vi "Cleanup.vi"(8 "error in (no error)":errorcluster, 11 "TCP_Streamer_Subscriber in":refnum<class "TCP_Streamer_Subscriber.lvclass">) -> (0 "error out":errorcluster, 3 "TCP_Streamer_Subscriber out":refnum<class "TCP_Streamer_Subscriber.lvclass">)   [LabVIEW 2021, in "TCP_Streamer_Subscriber.lvclass"]
uses:
  TCP_Streamer_Subscriber.lvclass
  TCP_Streamer_Subscriber.lvclass/TCP_Streamer_Subscriber.ctl
  Typedef/State.ctl
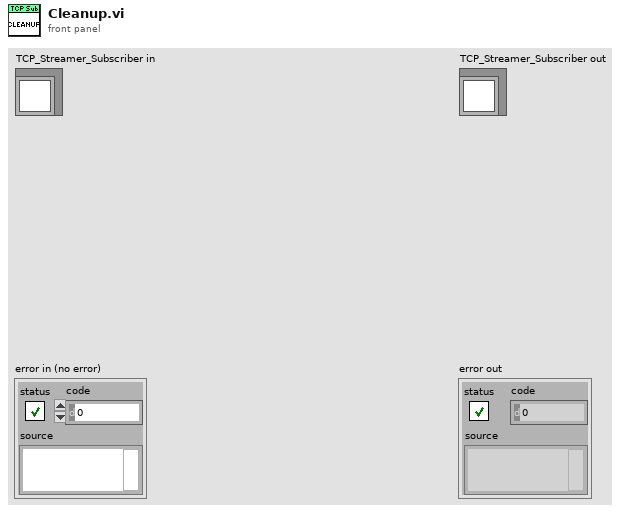
[diagram p1: front panel]
types:
  T1 = typedef "TCP_Streamer_Subscriber.lvclass/State.ctl" = enum16{"Stopped", "Connecting", "Receiving"}
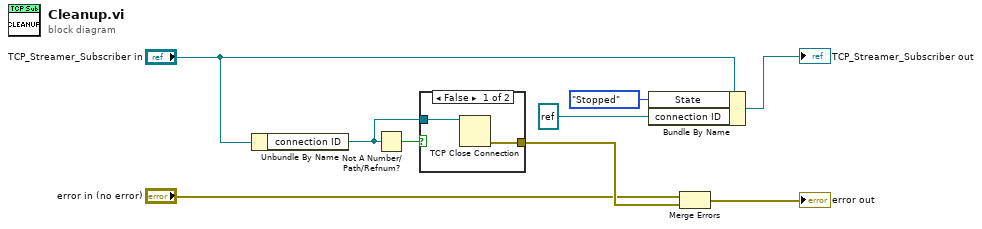
[diagram p0: block diagram]
diagram:
  n1 = Unbundle By Name("TCP_Streamer_Subscriber in") -> ("connection ID"=w4:refnum<k5>)
  n2 = Not A Number/Path/Refnum?(number/path/refnum=w4) -> (NaN/Path/Refnum?=w5:bool)
  n3 = case shown="False" w5 {
    tunnel: [w11 _] -> w8
    tunnel: w4 -> [w10 _]
    frame False {
      n4 = TCP Close Connection(connection ID=w10) -> (error out=w11:errorcluster)  [unwired: 2 in, 1 out]
    }
    frame True {
    }
  }
  n5 = Bundle By Name(cluster="TCP_Streamer_Subscriber in", "State"=State."Stopped", "connection ID"=refnum<k5> refnum) -> (→"TCP_Streamer_Subscriber out":refnum<class "TCP_Streamer_Subscriber.lvclass">)
  n6 = Merge Errors("error in (no error)", w8) -> (→"error out":errorcluster)
